vi "symmetry_v2.0.vi"() -> ()   [LabVIEW 2025]
doc: "Proof of concept/example VI for demonstration.\n\nMichael Panganiban\nSr. Hardware Test Engineer\nFresh Consulting, Inc."
panel:
  in  "Boolean 2":bool
  in  "Boolean":bool
  in  "Tab Control":T1(tab)
  in  "Enqueue Element":bool
  in  "stop":bool
  # "Fresh Consulting"
  # "v1.0.0.1"
  # "Running Test 1: Power ripple.."
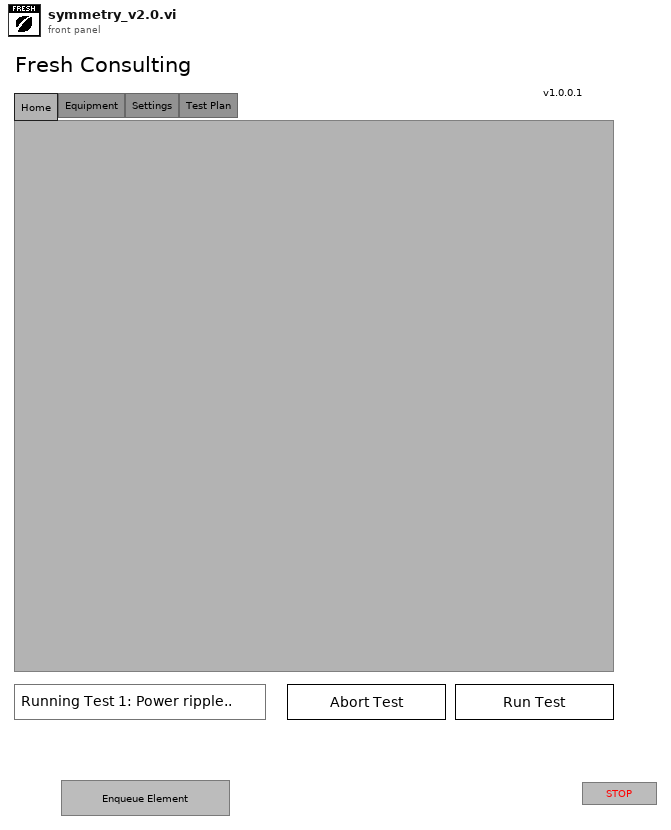
[diagram p1: front panel]
types:
  T1 = enum32{"Home", "Equipment", "Settings", "Test Plan"}
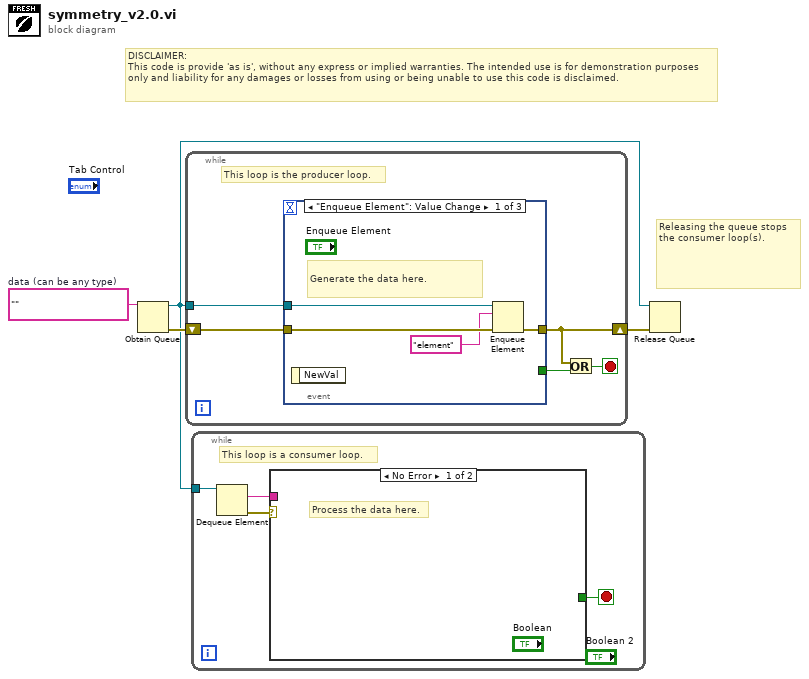
[diagram p0: block diagram]
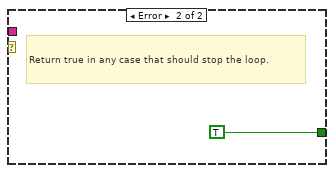
[diagram p2: hidden frame]
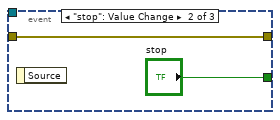
[diagram p3: hidden frame]
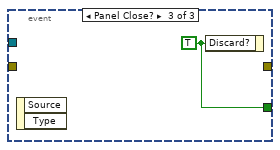
[diagram p4: hidden frame]
diagram:
  w2 = ""  # data (can be any type)
  # "DISCLAIMER:\nThis code is provide 'as is', without any express or implied warranties. The intended use is for demonstration purposes only and liability for any damages or losses from using or being unable to use this code is disclaimed."
  # "Releasing the queue stops the consumer loop(s)."
  n1 = Obtain Queue(element data type=w2) -> (queue out=w1:refnum<queue>, error out=w4:errorcluster)  [unwired: 4 in, 1 out]
  n2 = while {
    shift-right: [w5] -> w3
    shift-left: w4 -> [w8]
    tunnel: w1 -> [w9]
    stop <- w6 stop-if-true
    # "This loop is the producer loop."
    n3 = event shown="[0] \"Enqueue Element\": Value Change" {
      selector: _ -> [_ _ _]
      dyn-events: _ -> [_ _ _]
      timeout: _ -> [_ _ _]
      tunnel: w9 -> [w13 _ _]
      tunnel: w8 -> [w12 w14 _]
      tunnel: [w11 w14 _] -> w5
      tunnel: [_ "stop" w16] -> w7
      event "Enqueue Element": Value Change {
        # "Generate the data here."
        n4 = event-data() -> ()  [unwired: 1 in, 1 out]
        n5 = Enqueue Element(queue=w13, element="element", error in (no error)=w12) -> (error out=w11:errorcluster)  [unwired: 1 in, 2 out]
      }
      event "stop": Value Change {
        n6 = event-data() -> ()  [unwired: 1 in, 1 out]
      }
      event Panel Close? {
        w16 = TRUE ("Discard?")
        n7 = event-data() -> ()  [unwired: 1 in, 2 out]
        n8 = event-data("Discard?"=w16) -> ()  [unwired: 1 in, 1 out]
      }
    }
    n9 = Or(x=w5, y=w7) -> (x .or. y?=w6:bool)
  }
  n10 = while {
    tunnel: w1 -> [w20]
    stop <- w17 stop-if-true
    # "This loop is a consumer loop."
    n11 = Dequeue Element(queue=w20) -> (element=w18:string, error out=w19:errorcluster)  [unwired: 2 in, 2 out]
    n12 = case shown="No Error" w19 {
      tunnel: w18 -> [_ _]
      tunnel: [_ TRUE] -> w17
      frame No Error {
        # "Process the data here."
      }
      frame Error {
        # "Return true in any case that should stop the loop."
      }
    }
  }
  n13 = Release Queue(queue=w1, error in (no error)=w3) -> ()  [unwired: 1 in, 3 out]
